vi "Main_FGV_USE History.vi"(7 "Use Action":T2, 9 "Event":string, 10 "User Account Data":T3={"帳號 :"="", "權限等級："=enum."開發人員", "建立時間："="", "修改時間："="", "到期時間："="", "狀態："=enum."可使用", "期限："=enum."一天", "密碼："=""}, 11 "匯入硬體參數":path=path "D:/全域高斯機 參數/Paremeter") -> (3 "MSG Array":T1(array[cluster]))   [LabVIEW 2015]
uses:
  Use History.ctl
panel:
  out "error out":errorcluster
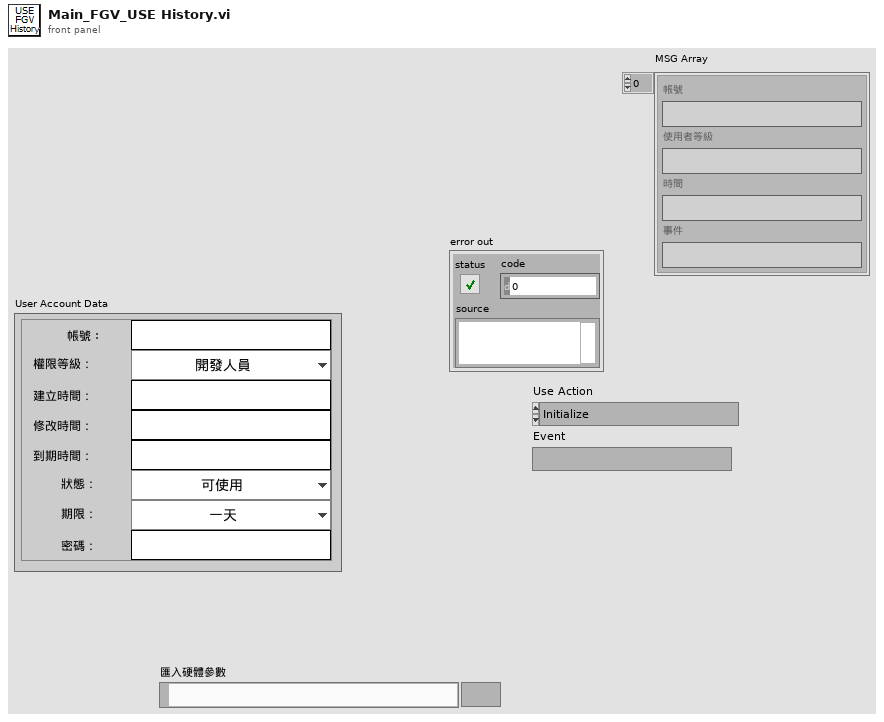
[diagram p1: front panel]
types:
  T1 = cluster{"帳號":string, "使用者等級":string, "時間":string, "事件":string}[]
  T2 = typedef "Use History.ctl" = enum16{"Initialize", "Set Data", "Get Data", "Idle"}
  T3 = typedef "Control_User account_Data.ctl" = cluster{"帳號 :":string, "權限等級：":T4, "建立時間：":string, "修改時間：":string, "到期時間：":string, "狀態：":T5, "期限：":T6, "密碼：":string}
  T4 = typedef "Control_User account_Permissions.ctl" = enum16{"開發人員", "管理者", "工程師", "作業員"}
  T5 = typedef "Control_User Accounts_Status.ctl" = enum16{"可使用", "不可使用"}
  T6 = typedef "Control_User account_Date.ctl" = enum16{"零天", "一天", "七天", "一個月", "一年", "三年"}
  T7 = cluster{"帳號 :":string, string, "date/time string":string, "Event":string}[]
  T8 = cluster{"帳號 :":string, string, "date/time string":string, "Event":string}
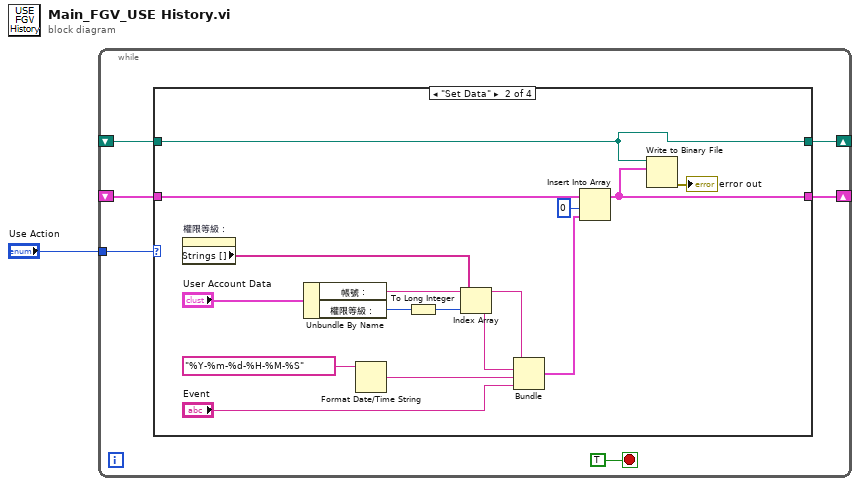
[diagram p0: block diagram]
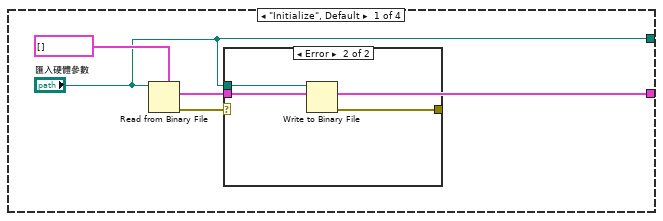
[diagram p2: hidden frame]
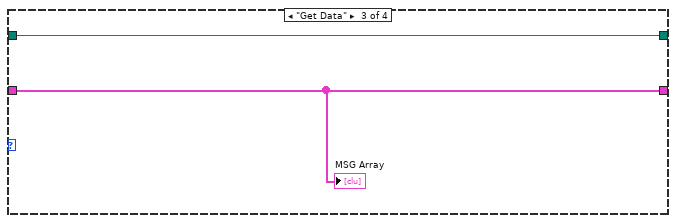
[diagram p4: hidden frame]
diagram:
  n1 = while {
    tunnel: "Use Action" -> [w6]
    shift-right: [w5] -> _
    shift-left: _ -> [w4]
    shift-right: [w3] -> _
    shift-left: _ -> [w2]
    stop <- TRUE stop-if-true
    n2 = case shown="\"Set Data\"" w6 {
      tunnel: [w9 w18 w31 w34] -> w5
      tunnel: w4 -> [_ w21 w31 w34]
      tunnel: ["匯入硬體參數" w17 w32 w33] -> w3
      tunnel: w2 -> [_ w17 w32 w33]
      frame "Initialize", Default {
        n3 = Read from Binary File(5:T7 [], 11:"匯入硬體參數") -> (0:w10:errorcluster, 2:w9:T7)  [unwired: 4 in, 2 out]
        n4 = case shown="Error" w10 {
          selector: w10 -> [w12 _]
          tunnel: "匯入硬體參數" -> [_ w15]
          tunnel: [w12 w14] -> _
          tunnel: w9 -> [_ w13]
          frame No Error {
          }
          frame Error {
            n5 = Write to Binary File(file (use dialog)=w15, data=w13) -> (error out=w14:errorcluster)  [unwired: 4 in, 2 out]
          }
        }
      }
      frame "Set Data" {
        n6 = property on="權限等級：" class="Enum (strict)"() -> ("Strings []"=w28:string[])  [unwired: 2 in, 2 out]
        n7 = Unbundle By Name("User Account Data") -> ("帳號 :"=w22:string, "權限等級："=w27:T4)
        n8 = Format Date/Time String(time format string (%c)="%Y-%m-%d-%H-%M-%S") -> (date/time string=w24:string)  [unwired: 2 in]
        n9 = To Long Integer(number=w27) -> (32bit integer=w26:i32)
        n10 = Index Array(array=w28, index=w26) -> (element=w25:string)
        n11 = Bundle("帳號 :"=w22, w25, "date/time string"=w24, "Event"="Event") -> (w20:T8)  [unwired: 1 in]
        n12 = Insert Into Array(array=w21, index=0, new element=w20) -> (w18:T7)
        n13 = Write to Binary File(file (use dialog)=w17, data=w18) -> (error out=→"error out":errorcluster)  [unwired: 4 in, 2 out]
      }
      frame "Get Data" {
        "MSG Array" <- w31
      }
      frame "Idle" {
      }
    }
  }
